vi "THz report connection.vi"(11 "THz MW generator constants":T1[](array[typedef])) -> (3 "string out":string)   [LabVIEW 2024, in "THz source modeule.lvlib"]
uses:
  THz source modeule.lvlib
  ctl/THz MW generator constants.ctl
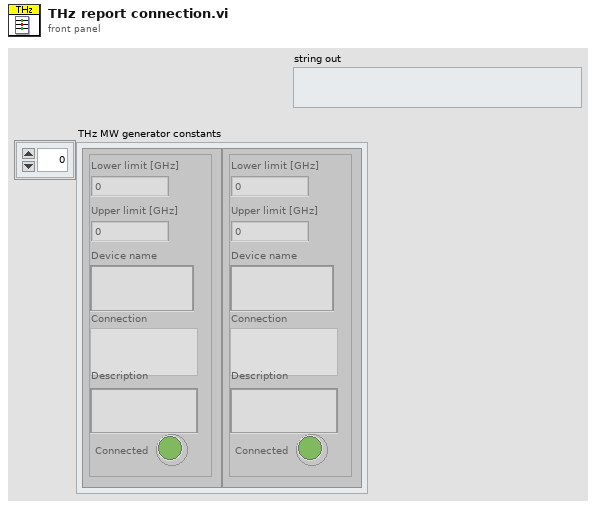
[diagram p1: front panel]
types:
  T1 = typedef "THz source modeule.lvlib/THz MW generator constants.ctl" = cluster{"Lower limit [GHz]":dbl, "Upper limit [GHz]":dbl, "Device name":string, "Connection":string, "Description":string, "Connected":bool}
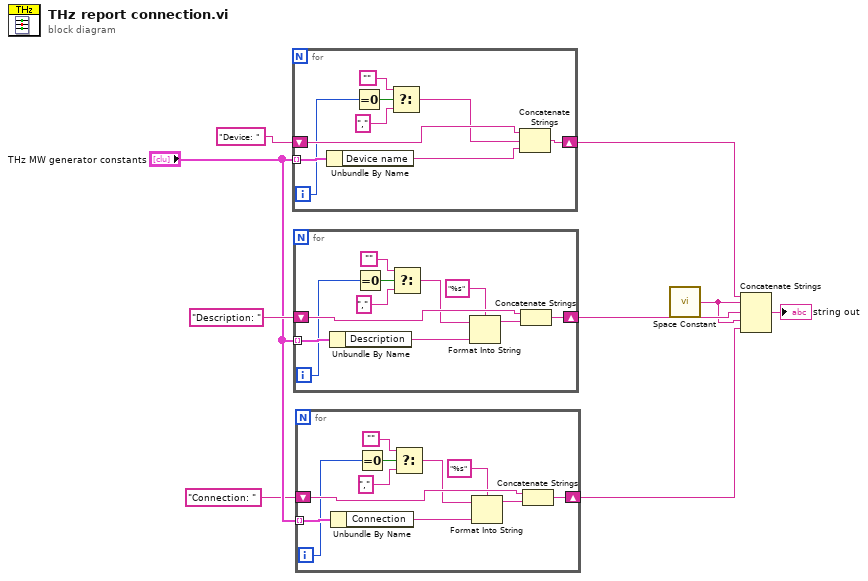
[diagram p0: block diagram]
diagram:
  n1 = for {
    tunnel: "THz MW generator constants" -> [w18] mode=indexing
    shift-right: [w16] -> w5
    shift-left: "Device: " -> [w17]
    i -> [w10]
    n2 = Unbundle By Name(w18) -> ("Device name"=w11:string)
    n3 = Equal To 0?(x=w10) -> (x = 0?=w15:bool)
    n4 = Select(t="", s=w15, f=",") -> (s? t:f=w12:string)
    n5 = Concatenate Strings(w17, w12, w11) -> (w16:string)
  }
  n6 = for {
    tunnel: "THz MW generator constants" -> [w29] mode=indexing
    shift-right: [w26] -> w4
    shift-left: "Description: " -> [w28]
    i -> [w19]
    n7 = Unbundle By Name(w29) -> ("Description"=w25:string)
    n8 = Equal To 0?(x=w19) -> (x = 0?=w23:bool)
    n9 = Select(t="", s=w23, f=",") -> (s? t:f=w22:string)
    n10 = Format Into String(format string="%s", initial string=w22, w25) -> (resulting string=w27:string)  [unwired: 1 in, 1 out]
    n11 = Concatenate Strings(w28, w27) -> (w26:string)
  }
  n12 = for {
    tunnel: "THz MW generator constants" -> [w40] mode=indexing
    shift-right: [w37] -> w2
    shift-left: "Connection: " -> [w39]
    i -> [w30]
    n13 = Unbundle By Name(w40) -> ("Connection"=w36:string)
    n14 = Equal To 0?(x=w30) -> (x = 0?=w34:bool)
    n15 = Select(t="", s=w34, f=",") -> (s? t:f=w33:string)
    n16 = Format Into String(format string="%s", initial string=w33, w36) -> (resulting string=w38:string)  [unwired: 1 in, 1 out]
    n17 = Concatenate Strings(w39, w38) -> (w37:string)
  }
  n18 = call <vilib>:"Space Constant.vi"() -> ("String"=w3:string)
  n19 = Concatenate Strings(w5, w3, w4, w3, w2) -> (→"string out":string)
